vi "Get Serial Number (Z).vi"(0 "VISA resource name in":refnum<visa-resource-name>, 3 "Error In":errorcluster) -> (7 "VISA resource name out":refnum<visa-resource-name>, 8 "Serial Number":u16, 9 "ACK":bool, 10 "Error out":errorcluster)   [LabVIEW 2015]
uses:
  Ctls/Cmd str.ctl
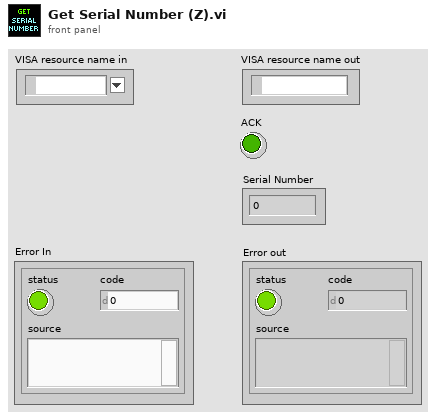
[diagram p1: front panel]
types:
  T1 = typedef "Cmd str.ctl" = string
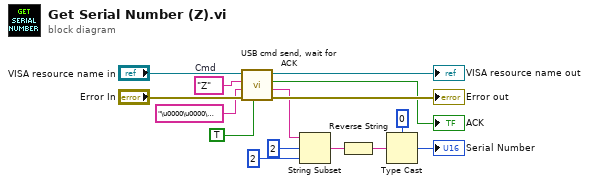
[diagram p0: block diagram]
diagram:
  w9 = T1 "Z"  # Cmd
  n1 = call "USB cmd send, wait for ACK.vi"("Wait for ACK?"=TRUE, "Error In"="Error In", "4 byte config str"="\u0000\u0000\u0000\u0000", "Cmd"=w9, "VISA resource name in"="VISA resource name in") -> ("Error out"=→"Error out":errorcluster, "Return msg"=w3:string, "ACK ok"=→"ACK":bool, "VISA resource name out"=→"VISA resource name out":refnum<visa-resource-name>)  [unwired: 1 in]
  n2 = String Subset(string=w3, offset (0)=2, length (rest)=2 ("length (rest)")) -> (substring=w6:string)
  n3 = Reverse String(1:w6) -> (0:w1:string)
  n4 = Type Cast(type=u16 0 ("offset (0)"), x=w1) -> (*(type *) &x=→"Serial Number":u16)
